vi "TCatAdsNetLibraryTester.vi"() -> ()   [LabVIEW 2016, in "TCatAdsNet.lvlib"]
uses:
  TCatAdsNet.lvlib
  AdsNET.lvclass
panel:
  out "Elapsed Time (ms)":u32
  out "Values (SGL)":sgl[](array[numeric])
  out "error out":errorcluster
  out "Value":string
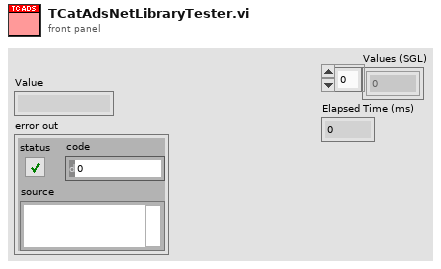
[diagram p1: front panel]
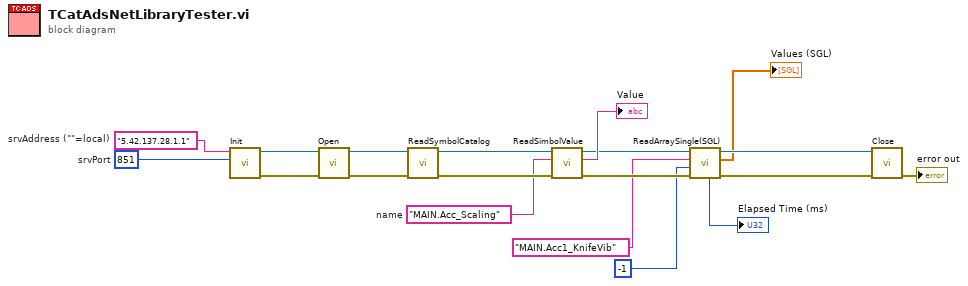
[diagram p0: block diagram]
diagram:
  w11 = "MAIN.Acc_Scaling"  # name
  w12 = 851  # srvPort
  w13 = "5.42.137.28.1.1"  # srvAddress (""=local)
  n1 = call "Init.vi"("srvPort"=w12, "srvAddress (\"\"=local)"=w13) -> ("error out"=w19:errorcluster, "TCatAdsNet"=w18:refnum<class "AdsNET.lvclass">)  [unwired: 8 in]
  n2 = call "Open.vi"("error in (no error)"=w19, "TCatAdsNet in"=w18) -> ("error out"=w17:errorcluster, "TCatAdsNet out"=w16:refnum<class "AdsNET.lvclass">)  [unwired: 8 in]
  n3 = call "ReadSymbolCatalog.vi"("error in (no error)"=w17, "AdsNET in"=w16) -> ("error out"=w14:errorcluster, "AdsNET out"=w15:refnum<class "AdsNET.lvclass">)  [unwired: 8 in]
  n4 = call "ReadSimbolValue.vi"("error in (no error)"=w14, "name"=w11, "TCatAdsNet in"=w15) -> ("error out"=w8:errorcluster, "Value"=→"Value":string, "TCatAdsNet out"=w6:refnum<class "AdsNET.lvclass">)  [unwired: 4 in, 2 out]
  n5 = call "ReadArraySingle(SGL).vi"("error in (no error)"=w8, "Elements (-1 = auto)"=-1, "variableName"="MAIN.Acc1_KnifeVib", "TCatAdsNet in"=w6) -> ("error out"=w7:errorcluster, "Values (SGL)"=→"Values (SGL)":sgl[], "TCatAdsNet out"=w5:refnum<class "AdsNET.lvclass">, "Elapsed Time (ms)"=→"Elapsed Time (ms)":u32)  [unwired: 3 in, 1 out]
  n6 = call "Close.vi"("error in (no error)"=w7, "TCatAdsNet in"=w5) -> ("error out"=→"error out":errorcluster)  [unwired: 9 in]
